vi "温湿度采集.vi"(11 "Modbus Master输入":refnum<class "Modbus Master.lvclass">) -> (1 "温度":string, 3 "湿度":string)   [LabVIEW 2020]
uses:
  <vilib>/NI/Modbus Library/API/Master/Modbus Master.lvclass
panel:
  out "湿度":dbl
  out "温度":dbl
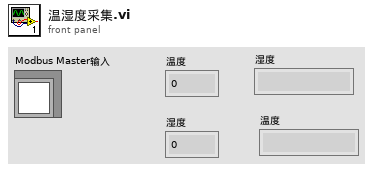
[diagram p1: front panel]
types:
  T1 = cluster{"地址":u16, "数量":u16, "寄存器值":u16[], "名称":string}[]
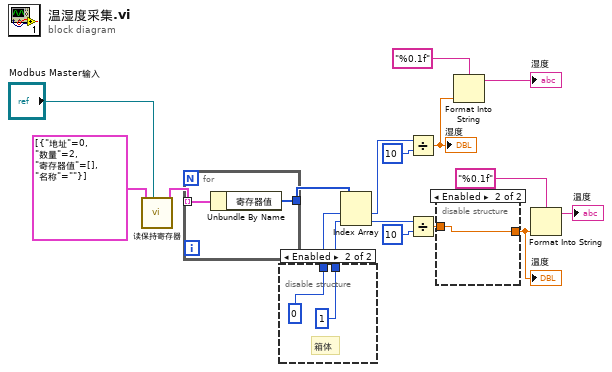
[diagram p0: block diagram]
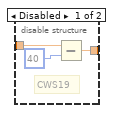
[diagram p2: hidden frame]
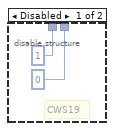
[diagram p3: hidden frame]
diagram:
  n1 = call "读保持寄存器.vi"("MB_实体"="Modbus Master输入", "读保持寄存器信息组__输入"=T1 [{"地址"=0, "数量"=2, "寄存器值"=[], "名称"=""}]) -> ("读保持寄存器信息组_输出"=w11:T1)  [unwired: 7 in, 2 out]
  n2 = for {
    tunnel: w11 -> [w19] mode=indexing
    tunnel: [w18] -> w14
    n3 = Unbundle By Name(w19) -> ("寄存器值"=w18:u16[])
  }
  n4 = disable-structure shown="Enabled" {
    disable-tunnel: [0 ("索引") 1 ("索引")] -> w15
    disable-tunnel: [1 ("索引") 0 ("索引")] -> w9
    frame Disabled {
      # "CWS19"
    }
    frame Enabled {
      # "箱体"
    }
  }
  n5 = Index Array(array=w14, index #1=w9, index #2=w15) -> (element #1=w2:u16, element #2=w1:u16)
  n6 = Divide(x=w2, y=u32 10) -> (x/y=w7:dbl)
  "湿度" <- w7
  n7 = Divide(x=w1, y=u32 10) -> (x/y=w16:dbl)
  n8 = disable-structure shown="Enabled" {
    disable-tunnel: w16 -> [w25 w27]
    disable-tunnel: [w24 w27] -> w5
    frame Disabled {
      # "CWS19"
      n9 = Subtract(x=w25, y=u32 40) -> (x-y=w24:dbl)
    }
    frame Enabled {
    }
  }
  "温度" <- w5
  n10 = Format Into String(format string="%0.1f" ("格式字符串"), w7) -> (resulting string=→"湿度":string)  [unwired: 2 in, 1 out]
  n11 = Format Into String(format string="%0.1f" ("格式字符串"), w5) -> (resulting string=→"温度":string)  [unwired: 2 in, 1 out]
